vi "update.path.vi"(8 "error in":errorcluster, 11 "Asset RID":string) -> (0 "error out":errorcluster, 2 "Path":string)   [LabVIEW 2020, in "asset.lvclass"]
uses:
  asset.lvclass
  asset.lvclass/asset.ctl
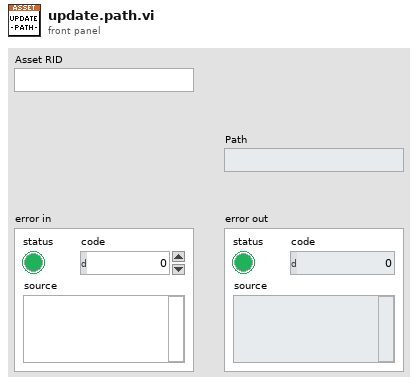
[diagram p1: front panel]
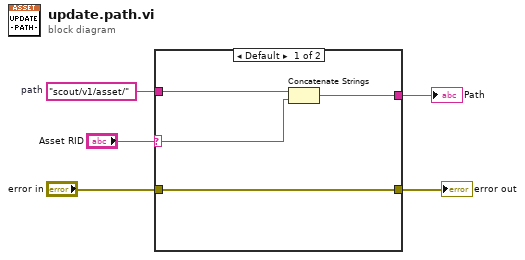
[diagram p0: block diagram]
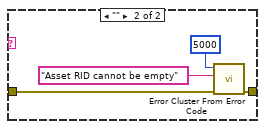
[diagram p2: hidden frame]
diagram:
  w5 = "scout/v1/asset/"  # path
  n1 = case shown="Default" "Asset RID" {
    selector: "Asset RID" -> [w8 _]
    tunnel: w5 -> [w9 _]
    tunnel: [w7 _] -> w3
    tunnel: [w6 w11] -> w1
    tunnel: "error in" -> [w6 w12]
    frame Default {
      n2 = Concatenate Strings(w9, w8) -> (w7:string)
    }
    frame "" {
      n3 = call <vilib>:"Error Cluster From Error Code.vi"("error in (no error)"=w12, "error message (\"\")"="Asset RID cannot be empty" ("error message (\"\")"), "error code (0)"=5000) -> ("error out"=w11:errorcluster)  [unwired: 6 in]
    }
  }
  "Path" <- w3
  "error out" <- w1
